vi "Password Authentication.vi"(8 "error in (no error)":errorcluster, 10 "Key":i16, 11 "Top Level in":refnum<class "Top Level.lvclass">) -> (0 "error out":errorcluster, 3 "Top Level out":refnum<class "Top Level.lvclass">)   [LabVIEW 2021, in "Top Level.lvlib" / "Top Level.lvclass"]
uses:
  Top Level.lvclass
  Top Level.lvclass/Top Level.ctl
  <vilib>/MGI/Panel Manager/Panel Actor/Panel Actor Messages/Show Panel Msg/Show Panel Msg.lvclass
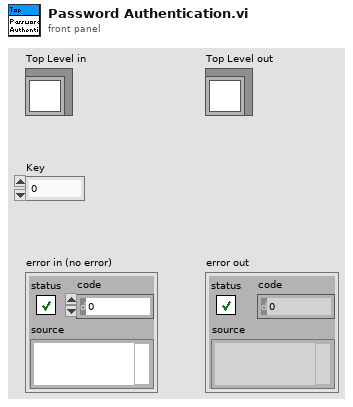
[diagram p1: front panel]
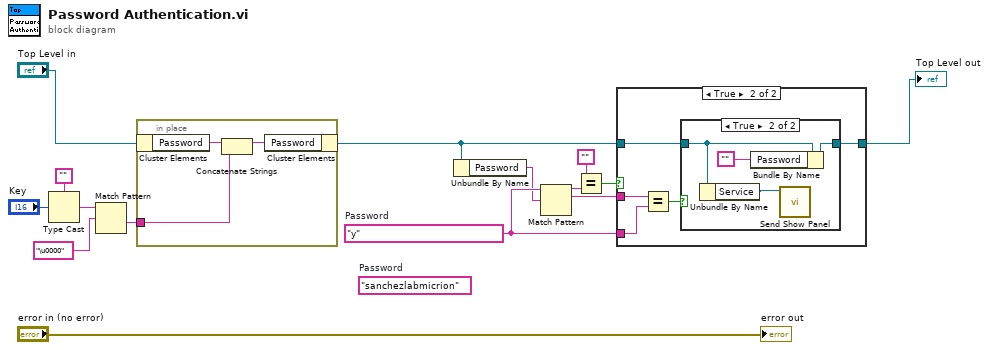
[diagram p0: block diagram]
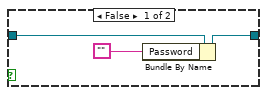
[diagram p2: hidden frame]
diagram:
  (unwired) "sanchezlabmicrion"  # Password
  w6 = "y"  # Password
  n1 = Type Cast(type="", x="Key") -> (*(type *) &x=w8:string)
  n2 = Match Pattern(string=w8, regular expression="\u0000") -> (after substring=w7:string)  [unwired: 1 in, 3 out]
  n3 = in-place {
    in-place-border: w7 -> [w16]
    n4 = in-place-cluster #1("Top Level in") -> ("Password"=w18:string)
    n5 = Concatenate Strings(w18, w16) -> (w17:string)
    n6 = in-place-cluster #1("Password"=w17) -> (w12:refnum<class "Top Level.lvclass">)
  }
  n7 = Unbundle By Name(w12) -> ("Password"=w5:string)
  n8 = Match Pattern(string=w6, regular expression=w5) -> (before substring=w4:string, match substring=w11:string)  [unwired: 1 in, 2 out]
  n9 = Equal?(x="", y=w4) -> (x = y?=w10:bool)
  n10 = case shown="True" w10 {
    tunnel: w12 -> [w21 w26]
    tunnel: [w20 w25] -> w1
    tunnel: w11 -> [_ w22]
    tunnel: w6 -> [_ w23]
    frame False {
      n11 = Bundle By Name(cluster=w21, "Password"="") -> (w20:refnum<class "Top Level.lvclass">)
    }
    frame True {
      n12 = Equal?(x=w22, y=w23) -> (x = y?=w24:bool)
      n13 = case shown="True" w24 {
        tunnel: w26 -> [w27 w28]
        tunnel: [w27 w30] -> w25
        frame False {
        }
        frame True {
          n14 = Unbundle By Name(w28) -> ("Service"=w31:refnum<class "Message Enqueuer.lvclass">)
          n15 = Bundle By Name(cluster=w28, "Password"="") -> (w30:refnum<class "Top Level.lvclass">)
          n16 = call <vilib>:"Send Show Panel.vi"("Message Enqueuer in"=w31) -> ()  [unwired: 9 in, 2 out]
        }
      }
    }
  }
  "Top Level out" <- w1
  "error out" <- "error in (no error)"
